vi "Format_DTU_RY.vi"() -> (2 "DTU2":string[](array[string]), 3 "DTU1":string[](array[string]))   [LabVIEW 2024, in "Keyence_VS150.lvlib"]
uses:
  Keyence_VS150.lvlib
  <userlib>/_OpenG.lib/string/string.llb/openg_string.lvlib
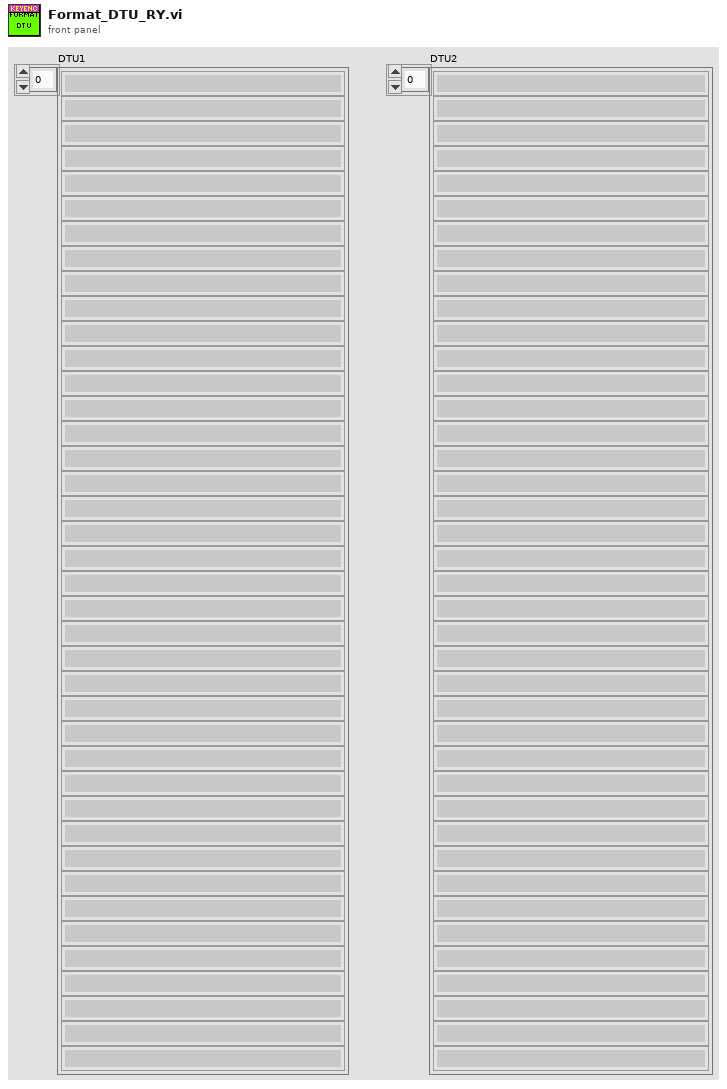
[diagram p1: front panel]
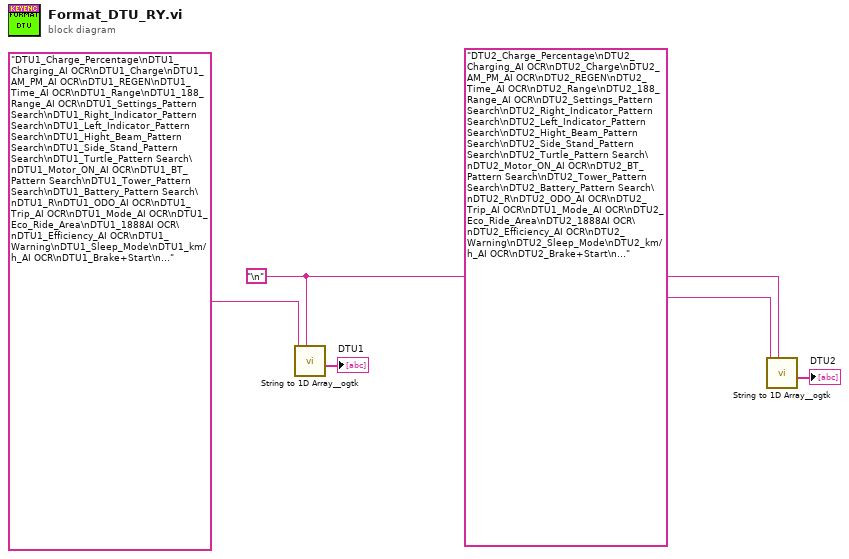
[diagram p0: block diagram]
diagram:
  w2 = "\n"
  n1 = call <userlib>:"String to 1D Array__ogtk.vi"("delimiter (Tab)"=w2, "string"="DTU1_Charge_Percentage\nDTU1_Charging_AI OCR\nDTU1_Charge\nDTU1_AM_PM_AI OCR\nDTU1_REGEN\nDTU1_Time_AI OCR\nDTU1_Range\nDTU1_188_Range_AI OCR\nDTU1_Settings_Pattern Search\nDTU1_Right_Indicator_Pattern Search\nDTU1_Left_Indicator_Pattern Search\nDTU1_Hight_Beam_Pattern Search\nDTU1_Side_Stand_Pattern Search\nDTU1_Turtle_Pattern Search\nDTU1_Motor_ON_AI OCR\nDTU1_BT_Pattern Search\nDTU1_Tower_Pattern Search\nDTU1_Battery_Pattern Search\nDTU1_R\nDTU1_ODO_AI OCR\nDTU1_Trip_AI OCR\nDTU1_Mode_AI OCR\nDTU1_Eco_Ride_Area\nDTU1_1888AI OCR\nDTU1_Efficiency_AI OCR\nDTU1_Warning\nDTU1_Sleep_Mode\nDTU1_km/h_AI OCR\nDTU1_Brake+Start\nDTU_Red_Area\nDTU1_Green_Area\nDTU1_Segment_Detection\nDTU1_White_Area" ("string (\"\")")) -> ("Array of Strings"=→"DTU1":string[])  [unwired: 9 in]
  n2 = call <userlib>:"String to 1D Array__ogtk.vi"("delimiter (Tab)"=w2, "string"="DTU2_Charge_Percentage\nDTU2_Charging_AI OCR\nDTU2_Charge\nDTU2_AM_PM_AI OCR\nDTU2_REGEN\nDTU2_Time_AI OCR\nDTU2_Range\nDTU2_188_Range_AI OCR\nDTU2_Settings_Pattern Search\nDTU2_Right_Indicator_Pattern Search\nDTU2_Left_Indicator_Pattern Search\nDTU2_Hight_Beam_Pattern Search\nDTU2_Side_Stand_Pattern Search\nDTU2_Turtle_Pattern Search\nDTU2_Motor_ON_AI OCR\nDTU2_BT_Pattern Search\nDTU2_Tower_Pattern Search\nDTU2_Battery_Pattern Search\nDTU2_R\nDTU2_ODO_AI OCR\nDTU2_Trip_AI OCR\nDTU1_Mode_AI OCR\nDTU2_Eco_Ride_Area\nDTU2_1888AI OCR\nDTU2_Efficiency_AI OCR\nDTU2_Warning\nDTU2_Sleep_Mode\nDTU2_km/h_AI OCR\nDTU2_Brake+Start\nDTU2_Red_Area\nDTU2_Green_Area\nDTU2_Segment_Detection\nDTU2_White_Area") -> ("Array of Strings"=→"DTU2":string[])  [unwired: 9 in]
